vi "_PC_Daemon_Config_Mass.vi"(6 "exe param memory":T1, 8 "error in (no error)":errorcluster) -> (0 "error out":errorcluster)   [LabVIEW 2018]
uses:
  <vilib>/event_ctls.llb/eventvkey.ctl
  PublicSubVI/Class/QMH/QMH.lvclass
panel:
  in  "ApplyBtn":bool
  in  "SetTab":enum32{"Execution", "Graph", "Communication"}(tab)
  in  "ContinuesRun":bool
  in  "Loops":i32=1 min=1
  in  "AVG":u8=1 min=1
  in  "Method":path
  in  "Width":u8[](array[numeric])=[1, 1, 1, 1, 1, 1, 1, 1, 1, 1] min=1 max=5
  in  "Color":u32[](array[colorbox])=[16860, 16711680, 1985280, 6618880, 15990570, 9567230, 8421568, 6946869, 0, 11796647]
  in  "BGColor":u32(colorbox)=16448250
  in  "XGrid":bool
  in  "YGrid":bool
  in  "Enable trigger start":bool
  in  "RS232 Trigger start":refnum<visa-resource-name>
  # "Loops :"
  # "AVG :"
  # "Continues Run :"
  # "BackGround Color :"
  # "Line Color :"
  # "Line Width :"
  # "X Grid :"
  # "Y Grid :"
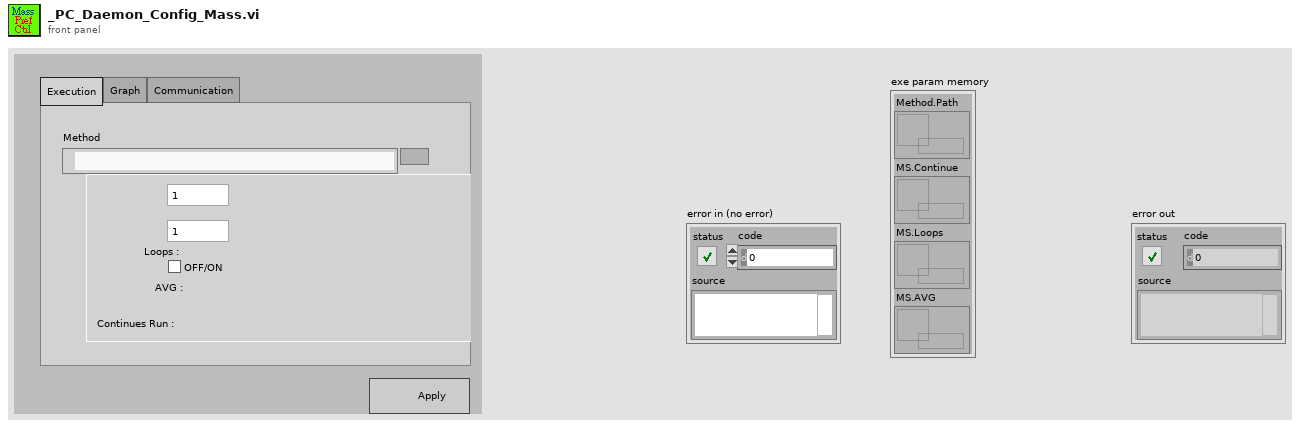
[diagram p1: front panel]
types:
  T1 = cluster{"Method.Path":refnum<data-value>, "MS.Continue":refnum<data-value>, "MS.Loops":refnum<data-value>, "MS.AVG":refnum<data-value>}
  T2 = enum32{"Invalid", "Default", "Floating", "Floating/Auto-Hide", "Modal"}
  T3 = enum16{"open", "replace", "create", "open or create", "replace or create", "replace or create with confirmation"}
  T4 = cluster{"BGColor":u32, "GridX":bool, "GridY":bool, "LineColorArray":u32[], "LineWidthArray":u8[]}
  T5 = cluster{"RS232 Trigger start":refnum<visa-resource-name>, "Enable trigger start":bool}
  T6 = cluster{"Method":path, "Loops":i32, "AVG":u8, "ContinuesRun":bool}
  T7 = typedef "eventvkey.ctl" = enum16{"ASCII", "Enter", "Return", "Shift", "Ctrl", "Alt", "Cmd", "Opt", "Caps", "NumLock", "Clear", "Break", "Up", "Down", "Left", "Right", "Insert", "Delete", "Home", "End", "PageUp", "PageDown", "Escape", "Help", "Pause", "ScrollLock", "F1", "F2", "F3", "F4", "F5", "F6", "F7", "F8", "F9", "F10", "F11", "F12", "F13", "F14", "F15", "F16", "F17", "F18", "F19", "F20", "F21", "F22", "F23", "F24", "Play", "VolumeUp", "VolumeDown", "Mute", "Two Byte Char"}
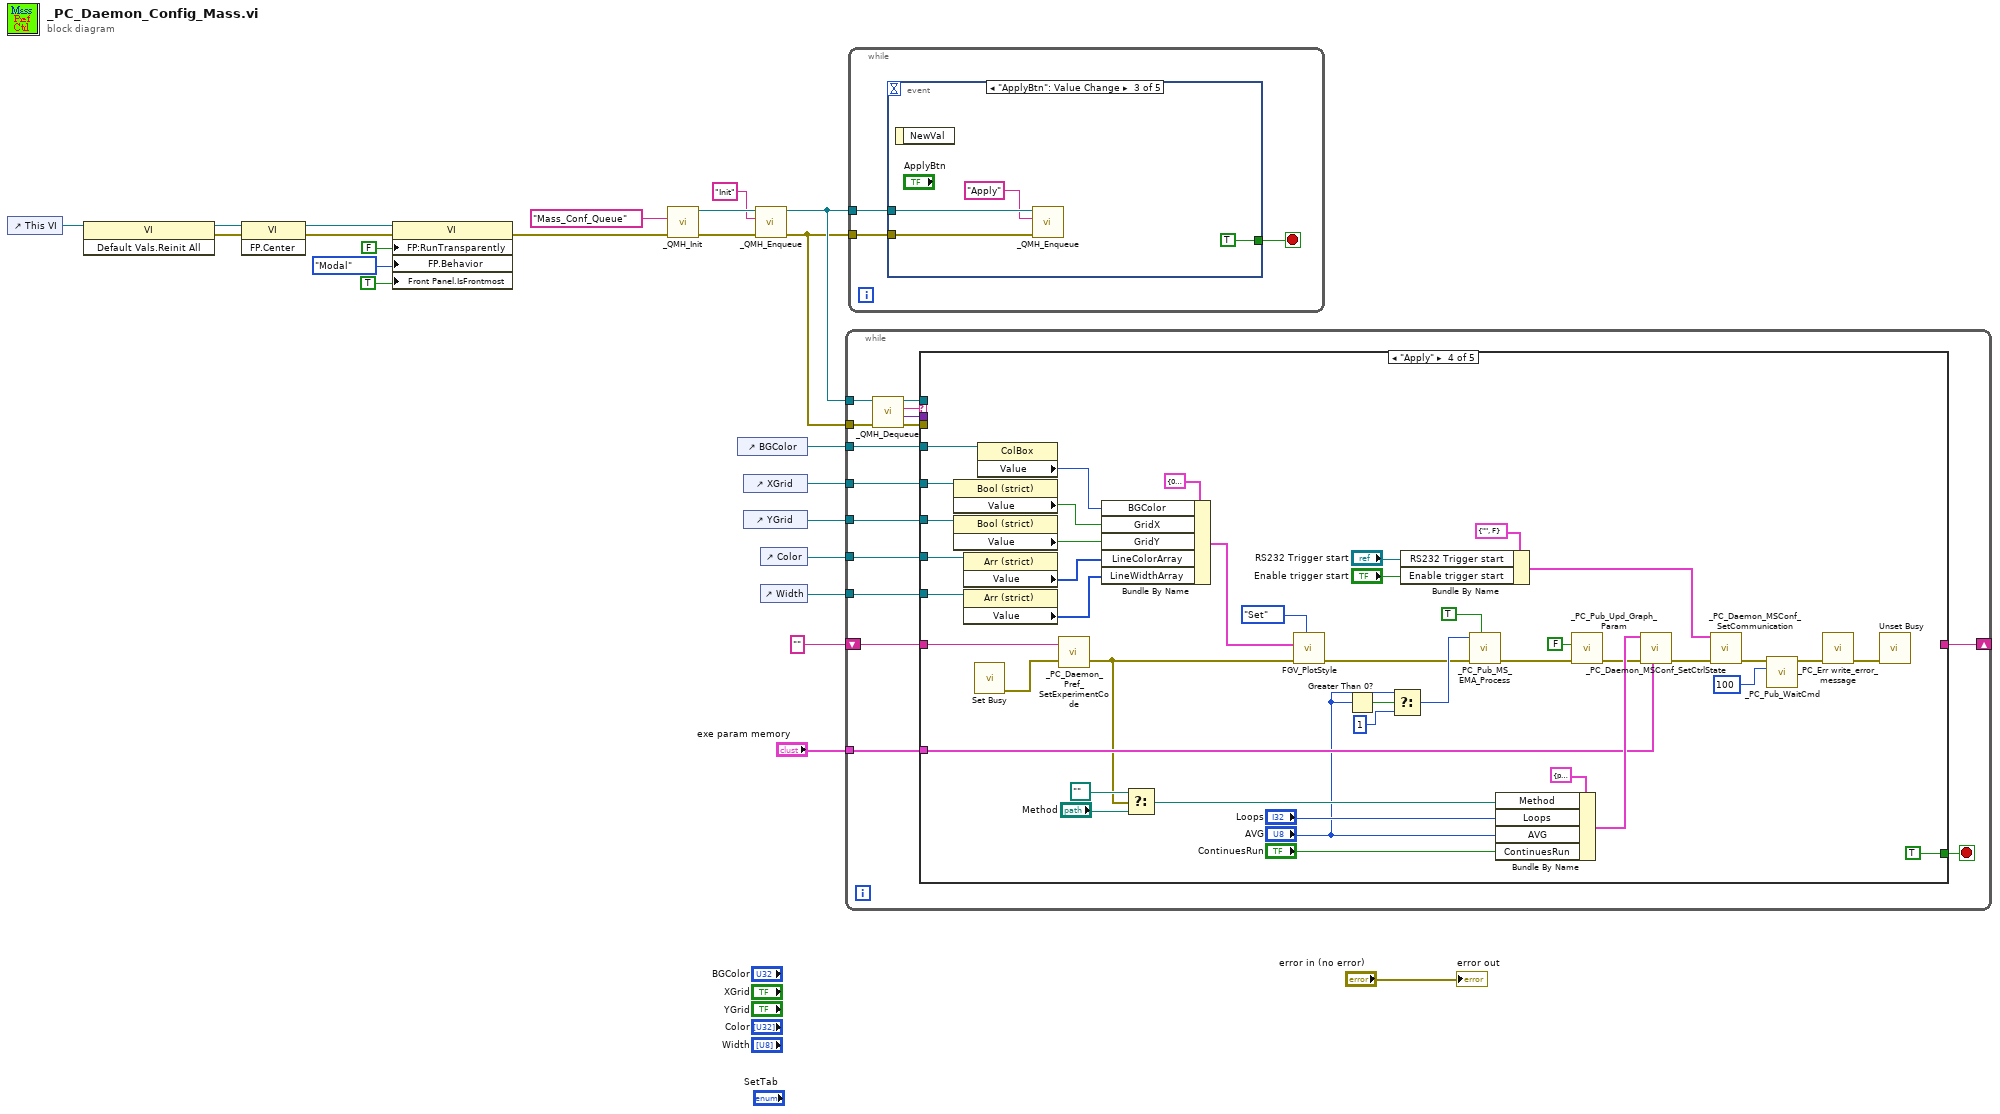
[diagram p0: block diagram]
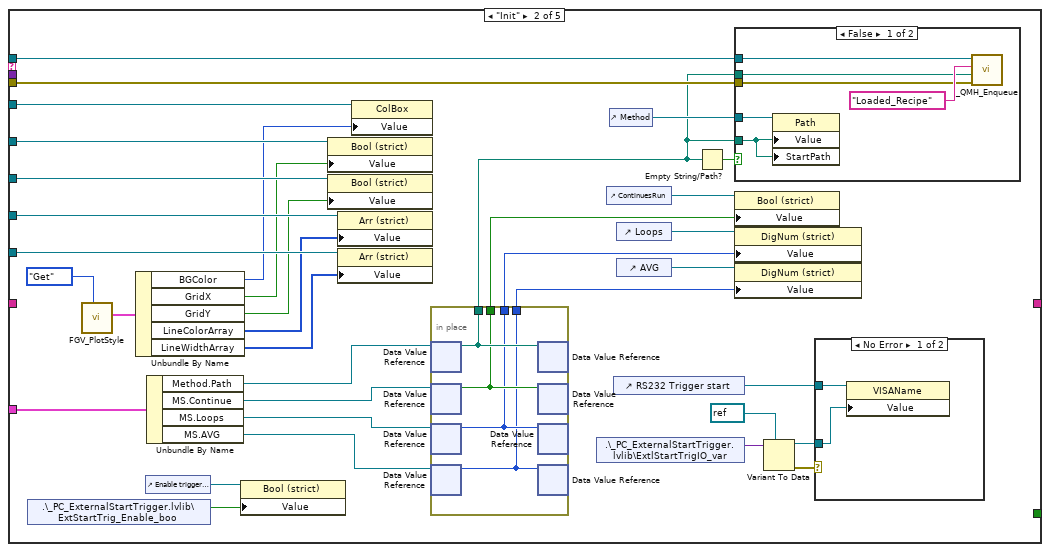
[diagram p3: hidden frame]
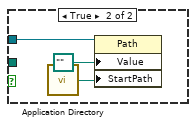
[diagram p4: hidden frame]
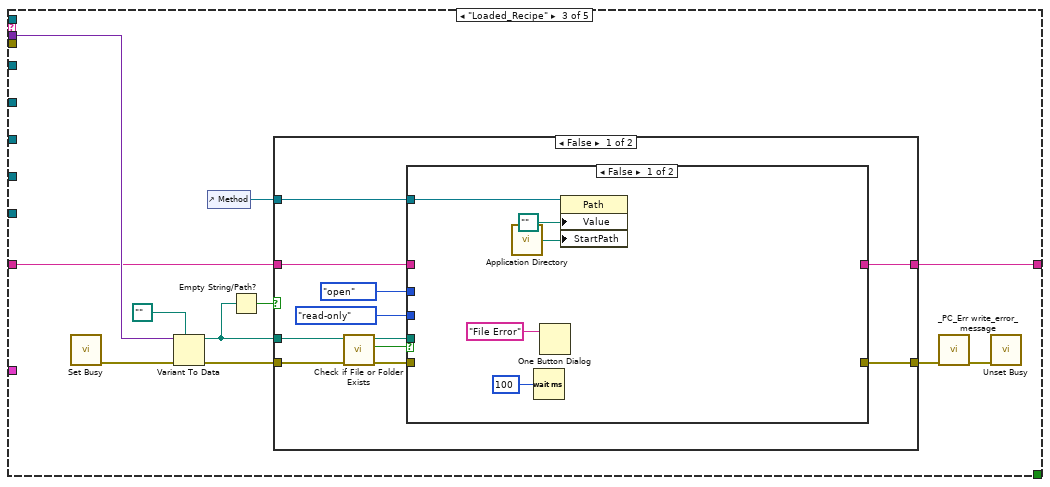
[diagram p6: hidden frame]
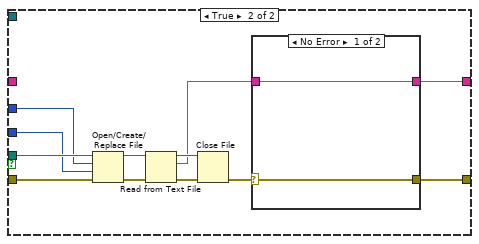
[diagram p7: hidden frame]
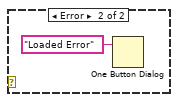
[diagram p8: hidden frame]
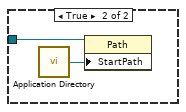
[diagram p9: hidden frame]
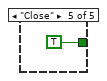
[diagram p10: hidden frame]
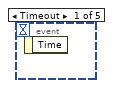
[diagram p11: hidden frame]
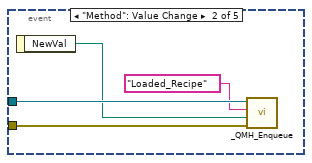
[diagram p12: hidden frame]
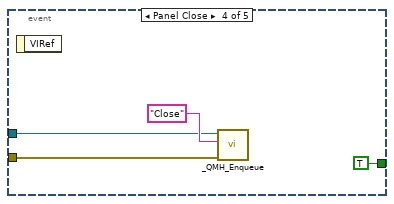
[diagram p13: hidden frame]
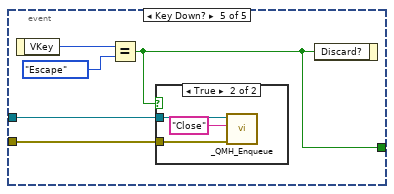
[diagram p14: hidden frame]
diagram:
  n1 = control-ref of="This VI"() -> (w5:refnum<vi>)
  n2 = invoke class="VI" method="Default Vals.Reinit All"(reference=w5) -> (reference out=w8:refnum<vi>, error out=w7:errorcluster)  [unwired: 2 in, 1 out]
  n3 = invoke class="VI" method="FP.Center"(reference=w8, error in=w7) -> (reference out=w9:refnum<vi>, error out=w6:errorcluster)  [unwired: 1 in, 1 out]
  n4 = property class="VI"(reference=w9, error in=w6, "FP:RunTransparently"=FALSE ("Front Panel Window:Run VI Transparently"), "FP.Behavior"=T2."Modal" ("Front Panel Window:Behavior"), "Front Panel.IsFrontmost"=TRUE ("Front Panel Window:Is Frontmost")) -> (error out=w4:errorcluster)  [unwired: 1 out]
  n5 = call "_QMH_Init.vi"("error in (no error)"=w4, "name (unnamed)"="Mass_Conf_Queue") -> ("error out"=w21:errorcluster, "QMH out"=w22:refnum<class "QMH.lvclass">)  [unwired: 8 in]
  n6 = control-ref of="BGColor"() -> (w17:refnum<vi>)
  n7 = control-ref of="XGrid"() -> (w16:refnum<vi>)
  n8 = control-ref of="YGrid"() -> (w15:refnum<vi>)
  n9 = call "_QMH_Enqueue.vi"("error in (no error)"=w21, "Msg"="Init", "QMH in"=w22) -> ("error out"=w18:errorcluster, "QMH out"=w19:refnum<class "QMH.lvclass">)  [unwired: 7 in]
  n10 = control-ref of="Color"() -> (w3:refnum<vi>)
  n11 = control-ref of="Width"() -> (w2:refnum<vi>)
  n12 = while {
    tunnel: w19 -> [w38]
    tunnel: w18 -> [w37]
    tunnel: w17 -> [w35]
    tunnel: w16 -> [w34]
    tunnel: w15 -> [w33]
    tunnel: w3 -> [w32]
    tunnel: w2 -> [w31]
    shift-right: [w28] -> _
    shift-left: "" -> [w29]
    tunnel: "exe param memory" -> [w24]
    stop <- w27 stop-if-true
    n13 = call "_QMH_Dequeue.vi"("error in (no error)"=w37, "QMH in"=w38) -> ("error out"=w25:errorcluster, "Data"=w30:variant, "Msg"=w36:string, "QMH out"=w26:refnum<class "QMH.lvclass">)  [unwired: 4 in, 2 out]
    n14 = case shown="\"Apply\"" w36 {
      tunnel: w35 -> [_ w74 _ w166 _]
      tunnel: w34 -> [_ w73 _ w165 _]
      tunnel: w33 -> [_ w72 _ w164 _]
      tunnel: w32 -> [_ w71 _ w163 _]
      tunnel: w31 -> [_ w70 _ w162 _]
      tunnel: w30 -> [_ _ w100 _ _]
      tunnel: w29 -> [w39 _ w97 w168 _]
      tunnel: [w39 _ w96 _ _] -> w28
      tunnel: [_ _ _ TRUE TRUE] -> w27
      tunnel: w26 -> [_ w54 _ _ _]
      tunnel: w25 -> [_ w53 _ _ _]
      tunnel: w24 -> [_ w49 _ w146 _]
      frame Default {
      }
      frame "Init" {
        n15 = shared-variable ".\\_PC_ExternalStartTrigger.lvlib\\ExtStartTrig_Enable_boo"() -> (w57:bool)  [unwired: 1 in, 1 out]
        n16 = call "FGV_PlotStyle.vi"("Function"=enum16{"Set", "Get"}."Get") -> ("Output Cluster"=w69:T4)  [unwired: 9 in, 1 out]
        n17 = Unbundle By Name(w69) -> ("BGColor"=w68:u32, "GridX"=w67:bool, "GridY"=w66:bool, "LineColorArray"=w65:u32[], "LineWidthArray"=w64:u8[])
        n18 = control-ref of="Enable trigger start"() -> (w63:refnum<vi>)
        n19 = Unbundle By Name(w49) -> ("Method.Path"=w48:refnum<data-value>, "MS.Continue"=w47:refnum<data-value>, "MS.Loops"=w46:refnum<data-value>, "MS.AVG"=w45:refnum<data-value>)
        n20 = property class="Bool (strict)"(reference=w63, "Value"=w57) -> ()  [unwired: 1 in, 2 out]
        n21 = property class="Bool (strict)"(reference=w73, "Value"=w67) -> ()  [unwired: 1 in, 2 out]
        n22 = property class="Bool (strict)"(reference=w72, "Value"=w66) -> ()  [unwired: 1 in, 2 out]
        n23 = property class="Arr (strict)"(reference=w71, "Value"=w65) -> ()  [unwired: 1 in, 2 out]
        n24 = property class="Arr (strict)"(reference=w70, "Value"=w64) -> ()  [unwired: 1 in, 2 out]
        n25 = property class="ColBox"(reference=w74, "Value"=w68) -> ()  [unwired: 1 in, 2 out]
        n26 = in-place {
          in-place-border: [w78] -> w44
          in-place-border: [w77] -> w40
          in-place-border: [w76] -> w43
          in-place-border: [w75] -> w41
          n27 = in-place-dvr #1(w48) -> (w78:path)  [unwired: 1 out]
          n28 = in-place-dvr #2(w47) -> (w77:bool)  [unwired: 1 out]
          n29 = in-place-dvr #3(w46) -> (w76:i32)  [unwired: 1 out]
          n30 = in-place-dvr #4(w45) -> (w75:u8)  [unwired: 1 out]
          n31 = in-place-dvr #1(w78) -> ()  [unwired: 2 out]
          n32 = in-place-dvr #2(w77) -> ()  [unwired: 2 out]
          n33 = in-place-dvr #3(w76) -> ()  [unwired: 2 out]
          n34 = in-place-dvr #4(w75) -> ()  [unwired: 2 out]
        }
        n35 = shared-variable ".\\_PC_ExternalStartTrigger.lvlib\\ExtlStartTrigIO_var"() -> (w58:variant)  [unwired: 1 in, 1 out]
        n36 = control-ref of="ContinuesRun"() -> (w42:refnum<vi>)
        n37 = control-ref of="Method"() -> (w51:refnum<vi>)
        n38 = control-ref of="RS232 Trigger start"() -> (w62:refnum<vi>)
        n39 = control-ref of="Loops"() -> (w55:refnum<vi>)
        n40 = control-ref of="AVG"() -> (w56:refnum<vi>)
        n41 = Empty String/Path?(string/path=w44) -> (empty?=w52:bool)
        n42 = case shown="False" w52 {
          tunnel: w54 -> [w83 _]
          tunnel: w53 -> [w82 _]
          tunnel: w44 -> [w81 _]
          tunnel: w51 -> [w80 w87]
          tunnel: w44 -> [w79 _]
          frame False {
            n43 = property class="Path"(reference=w80, "Value"=w79, "StartPath"=w79) -> ()  [unwired: 1 in, 2 out]
            n44 = call "_QMH_Enqueue.vi"("error in (no error)"=w82, "Data"=w81, "Msg"="Loaded_Recipe", "QMH in"=w83) -> ()  [unwired: 6 in, 2 out]
          }
          frame True {
            n45 = call <vilib>:"Application Directory.vi"() -> ("Application Directory"=w85:path)
            n46 = property class="Path"(reference=w87, "Value"=path "", "StartPath"=w85) -> ()  [unwired: 1 in, 2 out]
          }
        }
        n47 = property class="Bool (strict)"(reference=w42, "Value"=w40) -> ()  [unwired: 1 in, 2 out]
        n48 = property class="DigNum (strict)"(reference=w55, "Value"=w43) -> ()  [unwired: 1 in, 2 out]
        n49 = property class="DigNum (strict)"(reference=w56, "Value"=w41) -> ()  [unwired: 1 in, 2 out]
        n50 = Variant To Data(type=refnum<visa-resource-name> refnum ("NewVal"), Variant=w58) -> (data=w60:refnum<visa-resource-name>, error out=w61:errorcluster)  [unwired: 1 in]
        n51 = case shown="No Error" w61 {
          tunnel: w62 -> [w89 _]
          tunnel: w60 -> [w88 _]
          frame No Error {
            n52 = property class="VISAName"(reference=w89, "Value"=w88) -> ()  [unwired: 1 in, 2 out]
          }
          frame Error {
          }
        }
      }
      frame "Loaded_Recipe" {
        n53 = call <vilib>:"Set Busy.vi"() -> ("error out"=w95:errorcluster)  [unwired: 10 in, 1 out]
        n54 = Variant To Data(error in=w95, type=path "" ("path"), Variant=w100) -> (data=w93:path, error out=w98:errorcluster)
        n55 = control-ref of="Method"() -> (w94:refnum<vi>)
        n56 = Empty String/Path?(string/path=w93) -> (empty?=w92:bool)
        n57 = case shown="False" w92 {
          tunnel: w98 -> [w106 _]
          tunnel: w97 -> [w105 _]
          tunnel: [w104 _] -> w96
          tunnel: w93 -> [w103 _]
          tunnel: [w102 _] -> w91
          tunnel: w94 -> [w101 w133]
          frame False {
            n58 = call <vilib>:"Check if File or Folder Exists.vi"("error in (no error)"=w106, "path"=w103) -> ("error out"=w109:errorcluster, "file or folder exists?"=w111:bool, "dup path"=w110:path)  [unwired: 7 in]
            n59 = case shown="False" w111 {
              tunnel: w110 -> [_ w124]
              tunnel: w109 -> [_ w123]
              tunnel: T3."open" ("operation (0:open)") -> [_ w122]
              tunnel: enum16{"read/write", "read-only", "write-only"}."read-only" ("access (0:read/write)") -> [_ w121]
              tunnel: [_ w118] -> w104
              tunnel: w105 -> [_ _]
              tunnel: [_ w119] -> w102
              tunnel: w101 -> [w112 _]
              frame False {
                n60 = call <vilib>:"Application Directory.vi"() -> ("Application Directory"=w113:path)
                n61 = Wait (ms)(milliseconds to wait=u32 100) -> ()  [unwired: 1 out]
                n62 = One Button Dialog(message="File Error") -> ()  [unwired: 1 in, 1 out]
                n63 = property class="Path"(reference=w112, "Value"=path "", "StartPath"=w113) -> ()  [unwired: 1 in, 2 out]
              }
              frame True {
                n64 = Open/Create/Replace File(file path (use dialog)=w124, error in=w123, operation (0:open)=w122, access (0:read/write)=w121) -> (refnum out=w125:refnum<file>, error out=w126:errorcluster)  [unwired: 2 in, 1 out]
                n65 = Read from Text File(file (use dialog)=w125, error in=w126) -> (refnum out=w127:refnum<file>, text=w117:string, error out=w128:errorcluster)  [unwired: 2 in, 1 out]
                n66 = Close File(refnum=w127, error in=w128) -> (error out=w120:errorcluster)  [unwired: 1 out]
                n67 = case shown="No Error" w120 {
                  selector: w120 -> [w130 _]
                  tunnel: [w130 _] -> w119
                  tunnel: [w129 _] -> w118
                  tunnel: w117 -> [w129 _]
                  frame No Error {
                  }
                  frame Error {
                    n68 = One Button Dialog(message="Loaded Error") -> ()  [unwired: 1 in, 1 out]
                  }
                }
              }
            }
          }
          frame True {
            n69 = call <vilib>:"Application Directory.vi"() -> ("Application Directory"=w132:path)
            n70 = property class="Path"(reference=w133, "StartPath"=w132) -> ()  [unwired: 1 in, 2 out]
          }
        }
        n71 = call "_PC_Err write_error_message.vi"("error in"=w91) -> ("error out"=w90:errorcluster)  [unwired: 10 in]
        n72 = call <vilib>:"Unset Busy.vi"("error in (no error)"=w90) -> ()  [unwired: 10 in, 1 out]
      }
      frame "Apply" {
        n73 = property class="Bool (strict)"(reference=w165) -> ("Value"=w160:bool)  [unwired: 1 in, 2 out]
        n74 = property class="Bool (strict)"(reference=w164) -> ("Value"=w159:bool)  [unwired: 1 in, 2 out]
        n75 = property class="Arr (strict)"(reference=w163) -> ("Value"=w158:u32[])  [unwired: 1 in, 2 out]
        n76 = property class="Arr (strict)"(reference=w162) -> ("Value"=w157:u8[])  [unwired: 1 in, 2 out]
        n77 = call <vilib>:"Set Busy.vi"() -> ("error out"=w169:errorcluster)  [unwired: 10 in, 1 out]
        n78 = property class="ColBox"(reference=w166) -> ("Value"=w161:u32)  [unwired: 1 in, 2 out]
        n79 = call "_PC_Daemon_Pref_SetExperimentCode.vi"("error in (no error)"=w169, "FileData"=w168) -> ("error out"=w140:errorcluster)  [unwired: 1 in]
        n80 = Bundle By Name(cluster=T4 {"BGColor"=0, "GridX"=FALSE, "GridY"=FALSE, "LineColorArray"=[0, 0, 0, 0, 0, 0, 0, 0, 0, 0], "LineWidthArray"=[0, 0, 0, 0, 0, 0, 0, 1, 0, 0]} ("Input Cluster"), "BGColor"=w161, "GridX"=w160, "GridY"=w159, "LineColorArray"=w158, "LineWidthArray"=w157) -> (w144:T4)
        n81 = Select(t=path "", s=w140, f="Method") -> (s? t:f=w154:path)
        n82 = call "FGV_PlotStyle.vi"("Function"=enum16{"Set", "Get"}."Set", "error in (no error)"=w140, "Input Cluster"=w144) -> ("error out"=w135:errorcluster)  [unwired: 7 in, 1 out]
        n83 = Greater Than 0?(x="AVG") -> (x > 0?=w139:bool)
        n84 = Select(t="AVG", s=w139, f=u8 1) -> (s? t:f=w136:u8)
        n85 = Bundle By Name(cluster=T5 {"RS232 Trigger start"="", "Enable trigger start"=FALSE}, "RS232 Trigger start"="RS232 Trigger start", "Enable trigger start"="Enable trigger start") -> (w151:T5)
        n86 = call "_PC_Pub_MS_EMA_Process.vi"("Init? ( F )"=TRUE ("Init?"), "error in (no error)"=w135, "AVGValue"=w136) -> ("error out"=w134:errorcluster)  [unwired: 6 in, 2 out]
        n87 = Bundle By Name(cluster=T6 {"Method"=path "", "Loops"=1, "AVG"=1, "ContinuesRun"=FALSE}, "Method"=w154, "Loops"="Loops", "AVG"="AVG", "ContinuesRun"="ContinuesRun") -> (w156:T6)
        n88 = call "_PC_Pub_Upd_Graph_Param.vi"("error in (no error)"=w134, "Init?(F)"=FALSE) -> ("error out"=w152:errorcluster)  [unwired: 9 in]
        n89 = call "_PC_Daemon_MSConf_SetCtrlState.vi"("exe param memory"=w146, "error in (no error)"=w152, "Execution.Param"=w156) -> ("error out"=w145:errorcluster)  [unwired: 8 in]
        n90 = call "_PC_Daemon_MSConf_SetCommunication.vi"("error in (no error)"=w145, "Communication.Param"=w151) -> ("error out"=w150:errorcluster)  [unwired: 9 in]
        n91 = call "_PC_Pub_WaitCmd.vi"("milliseconds to wait"=u32 100, "error in (no error)"=w150) -> ("error out"=w149:errorcluster)  [unwired: 9 in]
        n92 = call "_PC_Err write_error_message.vi"("error in"=w149) -> ("error out"=w148:errorcluster)  [unwired: 10 in]
        n93 = call <vilib>:"Unset Busy.vi"("error in (no error)"=w148) -> ()  [unwired: 10 in, 1 out]
      }
      frame "Close" {
      }
    }
  }
  n94 = while {
    tunnel: w19 -> [w180]
    tunnel: w18 -> [w179]
    stop <- w178 stop-if-true
    n95 = event shown="[2] \"ApplyBtn\": Value Change" {
      selector: _ -> [_ _ _ _ _]
      dyn-events: _ -> [_ _ _ _ _]
      timeout: _ -> [_ _ _ _ _]
      tunnel: w180 -> [_ w184 w188 w190 w197]
      tunnel: w179 -> [_ w183 w187 w189 w196]
      tunnel: [_ _ TRUE TRUE w193] -> w178
      event Timeout {
        n96 = event-data() -> ()  [unwired: 1 in, 1 out]
      }
      event "Method": Value Change {
        n97 = event-data() -> ("NewVal"=w182:path)  [unwired: 1 in]
        n98 = call "_QMH_Enqueue.vi"("error in (no error)"=w183, "Data"=w182, "Msg"="Loaded_Recipe", "QMH in"=w184) -> ()  [unwired: 6 in, 2 out]
      }
      event "ApplyBtn": Value Change {
        n99 = event-data() -> ()  [unwired: 1 in, 1 out]
        n100 = call "_QMH_Enqueue.vi"("error in (no error)"=w187, "Msg"="Apply", "QMH in"=w188) -> ()  [unwired: 7 in, 2 out]
      }
      event Panel Close {
        n101 = event-data() -> ()  [unwired: 1 in, 1 out]
        n102 = call "_QMH_Enqueue.vi"("error in (no error)"=w189, "Msg"="Close", "QMH in"=w190) -> ()  [unwired: 7 in, 2 out]
      }
      event Key Down? {
        n103 = event-data() -> ("VKey"=w195:T7)  [unwired: 1 in]
        n104 = Equal?(x=w195, y=eventvkey."Escape") -> (x = y?=w193:bool)
        n105 = case shown="True" w193 {
          tunnel: w197 -> [_ w199]
          tunnel: w196 -> [_ w198]
          frame False {
          }
          frame True {
            n106 = call "_QMH_Enqueue.vi"("error in (no error)"=w198, "Msg"="Close", "QMH in"=w199) -> ()  [unwired: 7 in, 2 out]
          }
        }
        n107 = event-data("Discard?"=w193) -> ()  [unwired: 1 in, 1 out]
      }
    }
  }
  "error out" <- "error in (no error)"
